vi "Detect LabVIEW Versions.vi"() -> (2 "LabVIEW Versions":dbl[](array[numeric]))   [LabVIEW 2013]
doc: "Scans the National Instruments directory in Program Files (or (x86) on 64 bit) for LabVIEW installations and returns the version numbers for those found."
uses:
  <vilib>/Utility/sysdir.llb/System Directory Type.ctl
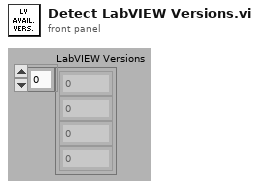
[diagram p1: front panel]
types:
  T1 = typedef "System Directory Type.ctl" = i32
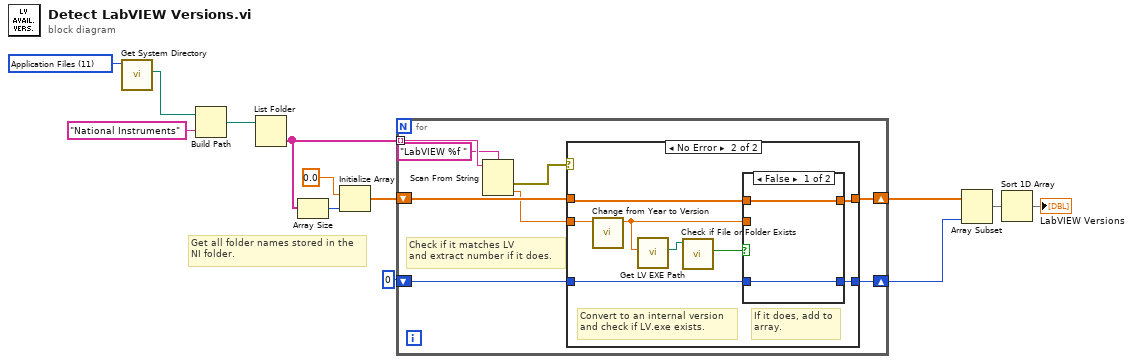
[diagram p0: block diagram]
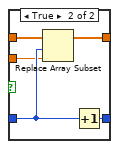
[diagram p3: hidden frame]
diagram:
  w13 = T1 11 items=["User Home"=0, "User Desktop"=1, "User Documents"=2, "User Application Data"=3, "User Preferences"=4, "User Temporary"=5, "Public Documents"=6, "Public Application Data"=7, "Public Preferences"=8, "Public Cache"=13, "System Core Libraries"=9, "System Installed Libraries"=10, "Application Files"=11, "Boot Volume Root"=12] ("system directory type")
  # "Get all folder names stored in the\nNI folder."
  n1 = call <vilib>:"Get System Directory.vi"("system directory type"=w13) -> ("system directory"=w12:path)  [unwired: 10 in]
  n2 = Build Path(base path=w12, name or relative path="National Instruments") -> (appended path=w10:path)
  n3 = List Folder(path=w10) -> (folder names=w6:string[])  [unwired: 3 in, 3 out]
  n4 = Array Size(array=w6) -> (size(s)=w9:i32)
  n5 = Initialize Array(0.0, w9) -> (w8:dbl[])
  n6 = for {
    tunnel: w6 -> [w17] mode=indexing
    shift-right: [w21] -> w5
    shift-left: w8 -> [w20]
    shift-right: [w19] -> w4
    shift-left: 0 -> [w18]
    # "Check if it matches LV\nand extract number if it does."
    n7 = Scan From String(format string="LabVIEW %f " ("regular expression"), input string=w17) -> (error out=w15:errorcluster, output 1=w14:dbl)  [unwired: 3 in, 2 out]
    n8 = case shown="No Error" w15 {
      tunnel: [w23 w30] -> w21
      tunnel: w20 -> [w23 w31]
      tunnel: [w22 w28] -> w19
      tunnel: w18 -> [w22 w29]
      tunnel: w14 -> [_ w27]
      frame Error {
      }
      frame No Error {
        # "If it does, add to\narray."
        # "Convert to an internal version\nand check if LV.exe exists."
        n9 = call "Change from Year to Version.vi"("LabVIEW Year"=w27) -> ("LabVIEW Version Number"=w26:dbl)  [unwired: 10 in]
        n10 = call "Get LV EXE Path.vi"("LabVIEW Version Number"=w26) -> ("appended path"=w25:path)  [unwired: 10 in]
        n11 = call <vilib>:"Check if File or Folder Exists.vi"("path"=w25) -> ("file or folder exists?"=w24:bool)  [unwired: 8 in, 2 out]
        n12 = case shown="False" w24 {
          tunnel: w31 -> [w33 w38]
          tunnel: [w33 w37] -> w30
          tunnel: w29 -> [w32 w36]
          tunnel: [w32 w35] -> w28
          tunnel: w26 -> [_ w34]
          frame False {
          }
          frame True {
            n13 = Replace Array Subset(array=w38, new element=w34, index=w36) -> (w37:dbl[])
            n14 = Increment(x=w36) -> (x+1=w35:i32)
          }
        }
      }
    }
  }
  n15 = Array Subset(array=w5, length=w4) -> (w2:dbl[])  [unwired: 1 in]
  n16 = Sort 1D Array(array=w2) -> (sorted array=→"LabVIEW Versions":dbl[])
